vi "过程变量.vi"() -> ()   [LabVIEW 2016, in "NAQ_DO.lvlib"]
uses:
  NAQ_DO.lvlib
panel:
  out "通讯状态":errorcluster
  out "检测值":T1
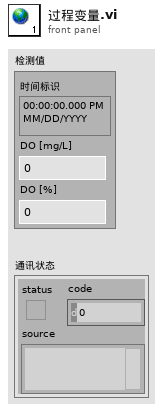
[diagram p1: front panel]
types:
  T1 = cluster{"时间标识":timestamp, "DO [mg/L]":dbl, "DO [%]":dbl}
diagram:
